vi "SigProc_method formatSignalData.vi"(7 "xLabelName":string, 8 "error in (no error)":errorcluster, 11 "spectraSignal":waveform(sgl)[](array[waveform])) -> (0 "error out":errorcluster, 3 "spectraData":cluster{"X":dbl[], "Y":sgl[]}[](array[cluster]), 5 "beta":dbl[](array[numeric]))   [LabVIEW 2018, in "Sig2MS.lvclass"]
uses:
  Sig2MS.lvclass
  SigInfo/SigInfo.lvclass
  DataXML/DataXML.lvclass
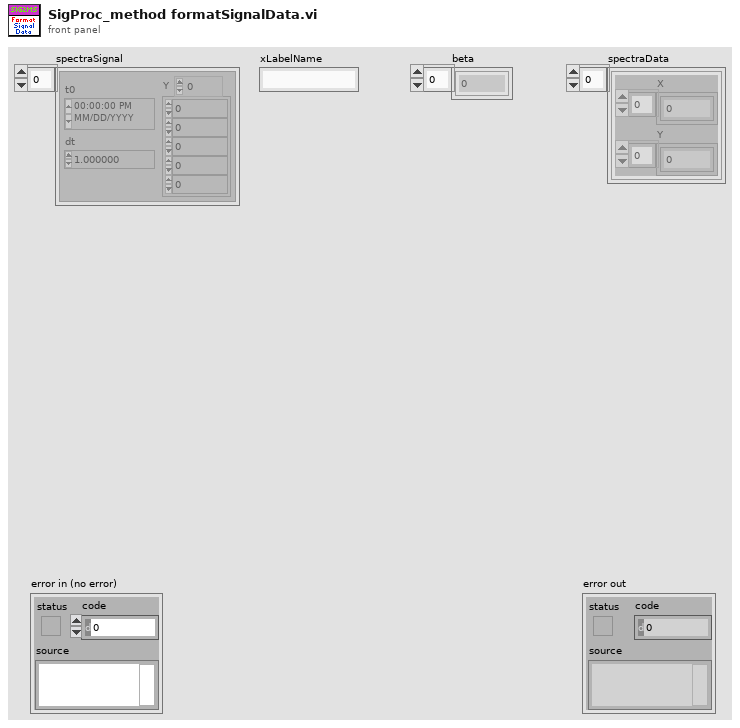
[diagram p1: front panel]
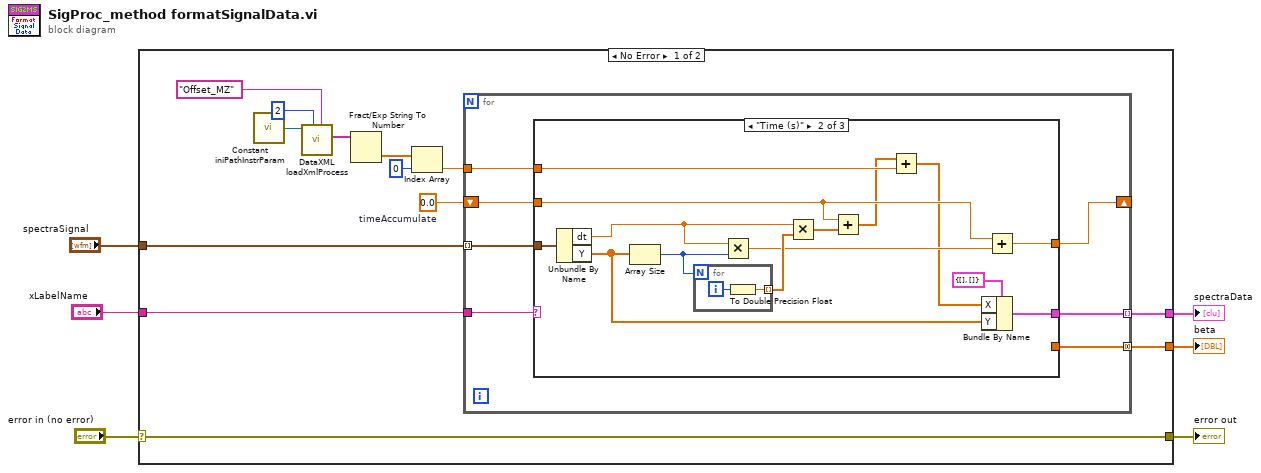
[diagram p0: block diagram]
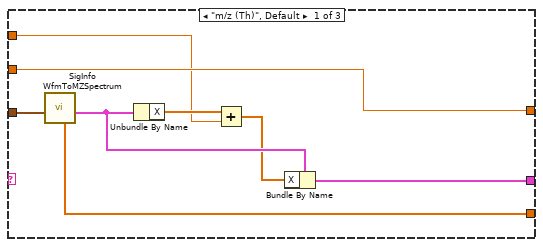
[diagram p2: hidden frame]
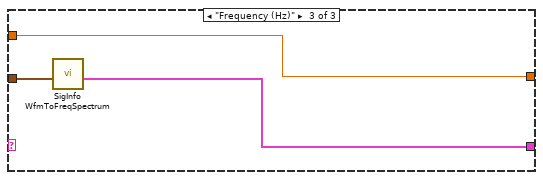
[diagram p3: hidden frame]
diagram:
  n1 = case shown="No Error" "error in (no error)" {
    selector: "error in (no error)" -> [w19 w54]
    tunnel: [w19 w54] -> w5
    tunnel: "spectraSignal" -> [w11 _]
    tunnel: [w10 _] -> w4
    tunnel: "xLabelName" -> [w9 _]
    tunnel: [w7 _] -> w2
    frame No Error {
      w8 = 0.0  # timeAccumulate
      n2 = call "Constant iniPathInstrParam.vi"() -> ("appended path"=w17:path)
      n3 = call "DataXML loadXmlProcess.vi"("target name"="Offset_MZ", "level"=u8 2, "xml_data_path"=w17) -> ("value"=w18:string[])  [unwired: 5 in, 3 out]
      n4 = Fract/Exp String To Number(string=w18) -> (number=w14:dbl[])  [unwired: 3 in, 1 out]
      n5 = Index Array(array=w14, index=0) -> (element=w12:dbl)
      n6 = for {
        tunnel: w12 -> [w26]
        tunnel: w11 -> [w25] mode=indexing
        tunnel: [w24] -> w10 mode=concatenating
        tunnel: w9 -> [w23]
        shift-right: [w21] -> _
        shift-left: w8 -> [w22]
        tunnel: [w20] -> w7 mode=indexing
        n7 = case shown="\"Time (s)\"" w23 {
          tunnel: w25 -> [w34 w48 w53]
          tunnel: w22 -> [w33 w38 w52]
          tunnel: [w33 w42 w52] -> w21
          tunnel: [w31 w39 w51] -> w20
          tunnel: w26 -> [w29 w37 _]
          tunnel: [w27 _ _] -> w24
          frame "m/z (Th)", Default {
            n8 = call "SigInfo WfmToMZSpectrum.vi"("SectionalSignal"=w34) -> ("MassSpectrum"=w32:cluster{"X":dbl[], "Y":sgl[]}, "beta"=w27:dbl[])  [unwired: 8 in, 1 out]
            n9 = Unbundle By Name(w32) -> ("X"=w30:dbl[])
            n10 = Add(x=w30, y=w29) -> (x+y=w28:dbl[])
            n11 = Bundle By Name(cluster=w32, "X"=w28) -> (w31:cluster{"X":dbl[], "Y":sgl[]})
          }
          frame "Time (s)" {
            n12 = Unbundle By Name(w48) -> ("dt"=w44:dbl, "Y"=w40:sgl[])
            n13 = Array Size(array=w40) -> (size(s)=w45:i32)
            n14 = for {
              N: w45 -> [_]
              tunnel: [w49] -> w47 mode=indexing
              i -> [w50]
              n15 = To Double Precision Float(number=w50) -> (double precision float=w49:dbl)
            }
            n16 = Multiply(x=w44, y=w45) -> (x*y=w43:dbl)
            n17 = Multiply(x=w44, y=w47) -> (x*y=w46:dbl[])
            n18 = Add(x=w38, y=w46) -> (x+y=w36:dbl[])
            n19 = Add(x=w36, y=w37) -> (x+y=w35:dbl[])
            n20 = Bundle By Name(cluster=cluster{"X":dbl[], "Y":sgl[]} {"X"=[], "Y"=[]} ("MassSpectrum"), "X"=w35, "Y"=w40) -> (w39:cluster{"X":dbl[], "Y":sgl[]})
            n21 = Add(x=w38, y=w43) -> (x+y=w42:dbl)
          }
          frame "Frequency (Hz)" {
            n22 = call "SigInfo WfmToFreqSpectrum.vi"("SectionalSignal"=w53) -> ("MassSpectrum"=w51:cluster{"X":dbl[], "Y":sgl[]})  [unwired: 9 in, 1 out]
          }
        }
      }
    }
    frame Error {
    }
  }
  "error out" <- w5
  "beta" <- w4
  "spectraData" <- w2
